vi "Stop.vi"(8 "error in (no error)":errorcluster, 11 "MQTT_Base in":refnum<class "MQTT_Base.lvclass">) -> (0 "error out":errorcluster, 1 "timed out?":bool, 3 "MQTT_Base out":refnum<class "MQTT_Base.lvclass">)   [LabVIEW 2013, in "MQTT Base.lvlib" / "MQTT_Base.lvclass"]
uses:
  MQTT_Base.lvclass
  MQTT_Base.lvclass/MQTT_Base.ctl
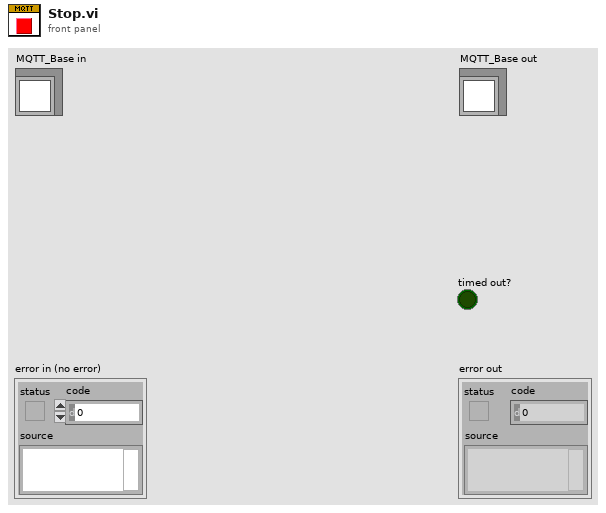
[diagram p1: front panel]
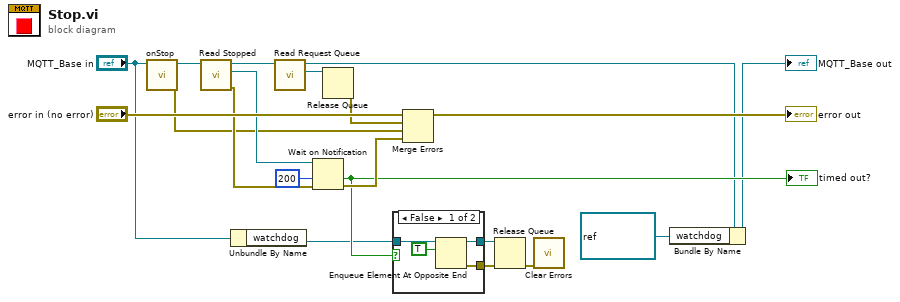
[diagram p0: block diagram]
diagram:
  n1 = call-dynamic "onStop.vi"("MQTT_Base in"="MQTT_Base in") -> ("error out"=w13:errorcluster, "MQTT_Base out"=w11:refnum<class "MQTT_Base.lvclass">)  [unwired: 9 in]
  n2 = call "Read Stopped.vi"("MQTT_Base in"=w11) -> ("error out"=w16:errorcluster, "Stopped"=w17:refnum<notifier>, "MQTT_Base out"=w10:refnum<class "MQTT_Base.lvclass">)  [unwired: 8 in]
  n3 = Unbundle By Name("MQTT_Base in") -> ("watchdog"=w5:refnum<queue>)
  n4 = call "Read Request Queue.vi"("MQTT_Base in"=w10) -> ("Request"=w15:refnum<queue>, "MQTT_Base out"=w4:refnum<class "MQTT_Base.lvclass">)  [unwired: 8 in, 1 out]
  n5 = Wait on Notification(notifier=w17, timeout in ms (-1)=200, error in (no error)=w16) -> (timed out?=w7:bool, error out=w12:errorcluster)  [unwired: 1 in, 2 out]
  "timed out?" <- w7
  n6 = Release Queue(queue=w15) -> (error out=w14:errorcluster)  [unwired: 2 in, 2 out]
  n7 = case shown="False" w7 {
    tunnel: w5 -> [w24 w25]
    tunnel: [w23 w25] -> w9
    tunnel: [w21 _] -> w8
    frame False {
      n8 = Enqueue Element At Opposite End(queue=w24, element=TRUE) -> (queue out=w23:refnum<queue>, error out=w21:errorcluster)  [unwired: 2 in, 1 out]
    }
    frame True {
    }
  }
  n9 = Merge Errors("error in (no error)", w14, w13, w12) -> (→"error out":errorcluster)
  n10 = Release Queue(queue=w9, error in (no error)=w8) -> (error out=w1:errorcluster)  [unwired: 1 in, 2 out]
  n11 = call <vilib>:"Clear Errors.vi"("error in (no error)"=w1) -> ()  [unwired: 6 in, 1 out]
  n12 = Bundle By Name(cluster=w4, "watchdog"=refnum<queue> refnum) -> (→"MQTT_Base out":refnum<class "MQTT_Base.lvclass">)
